vi "Lockin.Read Configuration File.vi"(8 "error in (no error)":errorcluster, 11 "Instrument.Lockin":refnum<class "Instrument.Lockin.lvclass">) -> (0 "error out":errorcluster, 3 "Instrument.Lockin out":refnum<class "Instrument.Lockin.lvclass">)   [LabVIEW 2016, in "Instrument.Lockin.lvclass"]
uses:
  Instrument.Lockin.lvclass
  C:/Program Files (x86)/National Instruments/LabVIEW 2016/user.lib/LevyLab/Levylab Instruments/SMOs/Instrument/Instrument.lvclass
  Instrument.Lockin.lvclass/Instrument.Lockin.ctl
  <userlib>/LevyLab/Levylab Instruments/SMOs/Instrument/Instrument.lvclass/Instrument.ctl
  <userlib>/LevyLab/Levylab Instruments/SMOs/Configuration/Configuration.lvclass
  <userlib>/LevyLab/Levylab Instruments/SMOs/Instrument/Instrument.lvclass
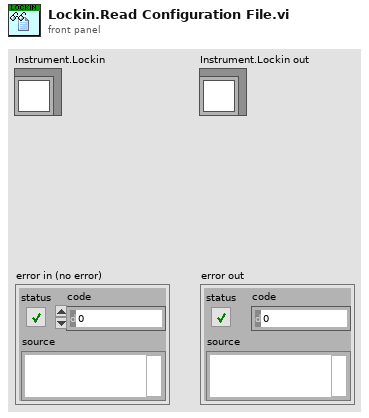
[diagram p1: front panel]
types:
  T1 = typedef "Instrument.Lockin.lvclass/Lockin.Configuration--Cluster.ctl" = cluster{"Channels: AO":T2, "Channels: REF":T4, "REF Filter":T5, "Amplifers":cluster{"offsets":dbl[], "Gain":dbl[], "Amplifiers":T6}, "DAQ":cluster{"sampling":T7, "sample mode":i32, "buffer size (S)":u32, "decimation":u32}, "Calibration":cluster{"Cal Info":T8[]}, "AI Configuration":T9, "AO Configuration":T14, "Aux Channel":tag}
  T2 = typedef "LockinDAQ.lvclass/AO-cluster.ctl" = cluster{"Ch":i32[], "Amp (V)":dbl[], "DC (V)":dbl[], "f (Hz)":dbl[], "Phase (°)":dbl[], "Function":T3[], "Sweep?":bool[]}
  T3 = typedef "LockinDAQ.lvclass/Function-enum.ctl" = enum16{"Sine", "Triangle", "Square", "Sawtooth"}
  T4 = typedef "LockinDAQ.lvclass/REF-cluster.ctl" = cluster{"Ch":i32[], " f (Hz)":dbl[], "Phase (°)":dbl[], "TC (s)":dbl[], "order":i32[]}
  T5 = typedef "LockinDAQ.lvclass/AI Prefilter-cluster.ctl" = cluster{"60 Hz prefilter":bool, "LP prefilter":bool, "LP cutoff (Hz)":dbl}
  T6 = typedef "LockinDAQ.lvclass/AmplifierType-enum.ctl" = enum16{"Manual", "Krohn Hite", "Femto"}
  T7 = typedef "LockinDAQ.lvclass/Sampling.ctl" = cluster{"Fs":dbl, "#s":i32}
  T8 = typedef "LockinDAQ.lvclass/Cal Info - Cluster.ctl" = cluster{"Active Device":tag, "SelfCal.LastDate/Time":timestamp, "SelfCal.LastTemp":dbl, "DevTemp":dbl, "calibration due?":bool}
  T9 = typedef "LockinDAQ.lvclass/AI.config-array.ctl" = T10[]
  T10 = typedef "LockinDAQ.lvclass/AI.config-cluster.ctl" = cluster{"AI.channels":tag, "AI.Coupling":T11, "AI.Range":T12, "input terminal configuration":i32, "DAQ Type":T13}
  T11 = typedef "LockinDAQ.lvclass/AI.coupling-enum.ctl" = u16
  T12 = typedef "LockinDAQ.lvclass/446xAI-enum.ctl" = enum16{"±0.316 V", "±1.00 V", "±3.16 V", "±10.0 V", "±31.6 V", "±42.4 V"}
  T13 = typedef "LockinDAQ.lvclass/DAQType-enum.ctl" = enum16{"None", "USB 4431", "PXI 446x"}
  T14 = typedef "LockinDAQ.lvclass/AO.config-array.ctl" = T15[]
  T15 = typedef "LockinDAQ.lvclass/AO.config-cluster.ctl" = cluster{"AO.channels":tag, "AO.Range":T16, "output terminal configuration":i32, "DAQ Type":T13}
  T16 = typedef "LockinDAQ.lvclass/446xAO-enum.ctl" = enum16{"±0.1 V", "±1.0 V", "±10.0 V"}
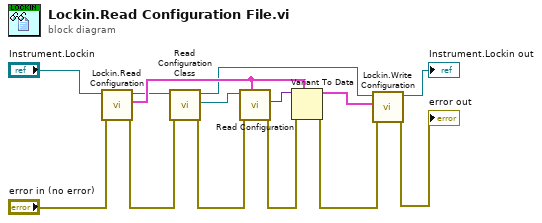
[diagram p0: block diagram]
diagram:
  n1 = call "Lockin.Read Configuration.vi"("error in (no error)"="error in (no error)", "Instrument.Lockin"="Instrument.Lockin") -> ("error out"=w6:errorcluster, "Configuration"=w10:T1, "Instrument.Lockin out"=w8:refnum<class "Instrument.Lockin.lvclass">)  [unwired: 7 in]
  n2 = call <userlib>:"Read Configuration Class.vi"("error in (no error)"=w6, "Instrument in"=w8) -> ("error out"=w5:errorcluster, "Configuration.lvclass"=w9:refnum<class "Configuration.lvclass">, "Instrument out"=w7:refnum<class "Instrument.Lockin.lvclass">)  [unwired: 7 in]
  n3 = call <userlib>:"Read Configuration.vi"("INI Fomatted Cluster Type"=w10, "error in (no error)"=w5, "Configuration in"=w9) -> ("error out"=w13:errorcluster, "Configuration"=w14:variant)  [unwired: 6 in, 1 out]
  n4 = Variant To Data(error in=w13, type=w10, Variant=w14) -> (data=w12:T1, error out=w11:errorcluster)
  n5 = call "Lockin.Write Configuration.vi"("error in (no error)"=w11, "Configuration"=w12, "Instrument.Lockin"=w7) -> ("error out"=→"error out":errorcluster, "Instrument.Lockin out"=→"Instrument.Lockin out":refnum<class "Instrument.Lockin.lvclass">)  [unwired: 7 in]
